vi "dark int time.vi"(8 "error in (no error)":errorcluster, 11 "Settings In":T1) -> (0 "error out":errorcluster, 1 "Stop and Save":bool, 3 "Settings Out":T1)   [LabVIEW 2014, in "AvaSpec.lvlib" / "Dark.lvlib"]
doc: "Determin the integration time to use for the next dark measurement based on how many dark measurements have already been taken and the configuration file."
uses:
  Dark.lvlib
  Settings/Settings.ctl
  Acquisition/Hardware Configuration.ctl
  Libraries/AS-5216-DLL/AVS settings.ctl
  Acquisition/Sphere Indicator.ctl
  Settings/Measurement Type.ctl
  Logging/Logging Configuration.ctl
  Settings/AvaSpec Settings.lvlib
  AvaSpec.lvlib
  Acquisition/AvaSpec Acquisition.lvlib
  Logging/AvaSpec Logging.lvlib
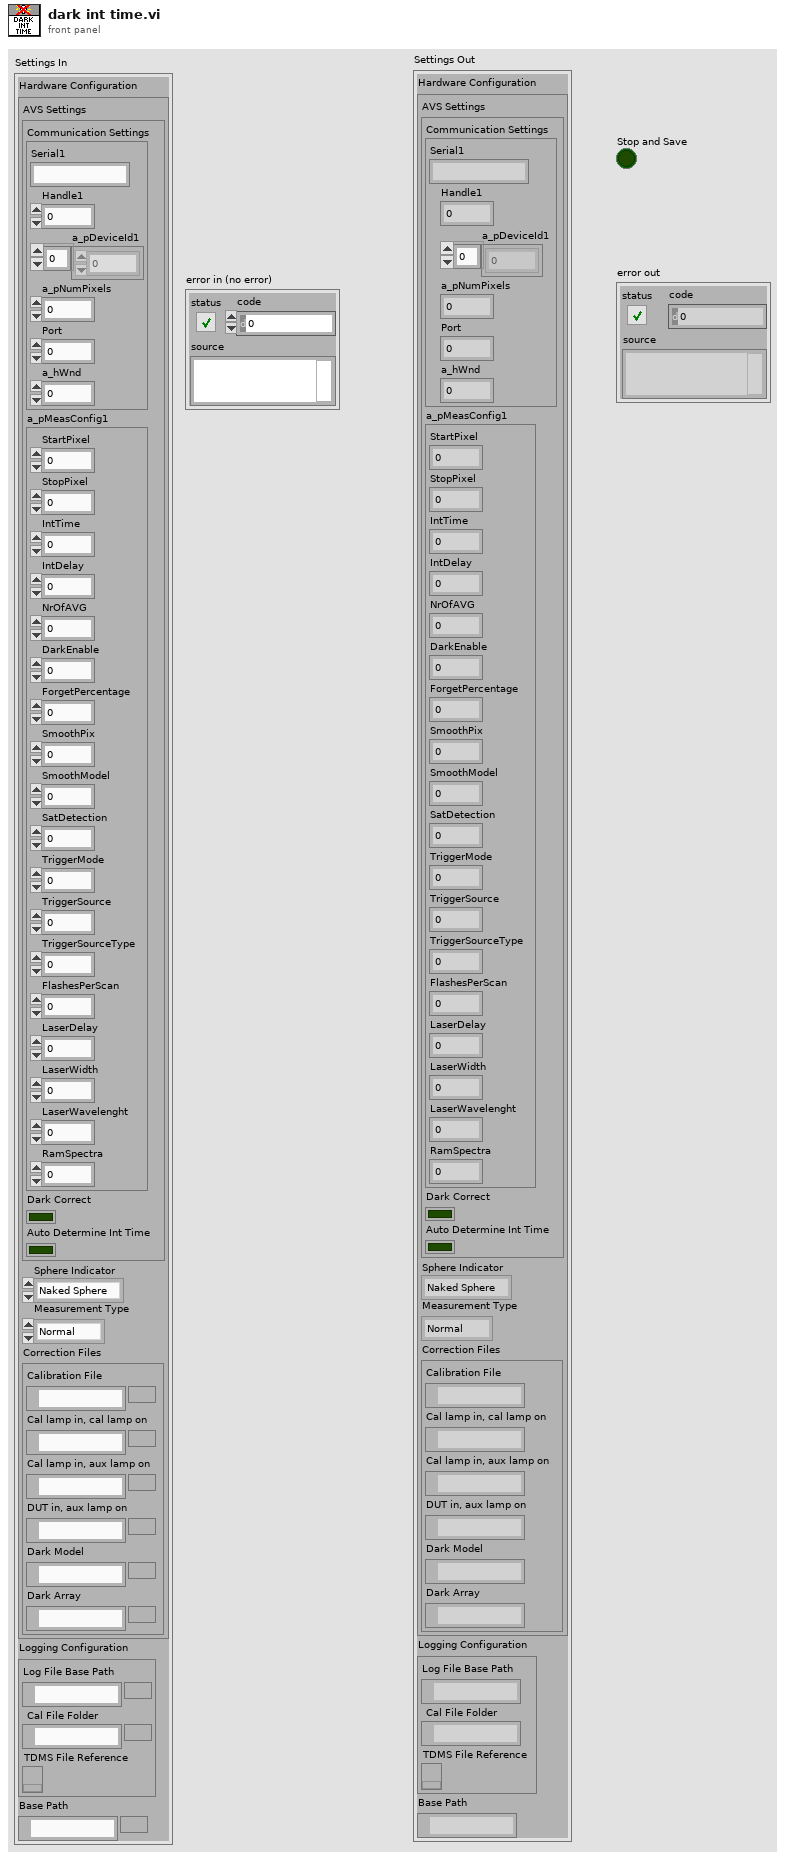
[diagram p1: front panel]
types:
  T1 = typedef "AvaSpec.lvlib/AvaSpec Settings.lvlib/Settings.ctl" = cluster{"Hardware Configuration":T2, "Logging Configuration":T6, "Base Path":path}
  T2 = typedef "AvaSpec.lvlib/AvaSpec Acquisition.lvlib/Hardware Configuration.ctl" = cluster{"AVS Settings":T3, "Sphere Indicator":T4, "Measurement Type":T5, "Correction Files":cluster{"Calibration File":path, "Cal lamp in, cal lamp on":path, "Cal lamp in, aux lamp on":path, "DUT in, aux lamp on":path, "Dark Model":path, "Dark Array":path}}
  T3 = typedef "AvaSpec.lvlib/AVS settings.ctl" = cluster{"Communication Settings":cluster{"Serial1":string, "Handle1":i32, "a_pDeviceId1":u8[], "a_pNumPixels":u16, "Port":i32, "a_hWnd":i32}, "a_pMeasConfig1":cluster{"StartPixel":u16, "StopPixel":u16, "IntTime":sgl, "IntDelay":u32, "NrOfAVG":u32, "DarkEnable":u8, "ForgetPercentage":u8, "SmoothPix":u16, "SmoothModel":u8, "SatDetection":u8, "TriggerMode":u8, "TriggerSource":u8, "TriggerSourceType":u8, "FlashesPerScan":u16, "LaserDelay":u32, "LaserWidth":u32, "LaserWavelenght":sgl, "RamSpectra":u16}, "Dark Correct":bool, "Auto Determine Int Time":bool}
  T4 = typedef "AvaSpec.lvlib/Sphere Indicator.ctl" = enum16{"Naked Sphere", "Insulated Sphere"}
  T5 = typedef "AvaSpec.lvlib/AvaSpec Acquisition.lvlib/Measurement Type.ctl" = enum16{"Normal", "Calibration", "Dark"}
  T6 = typedef "AvaSpec.lvlib/AvaSpec Logging.lvlib/Logging Configuration.ctl" = cluster{"Log File Base Path":path, "Cal File Folder":path, "TDMS File Reference":refnum<k34>}
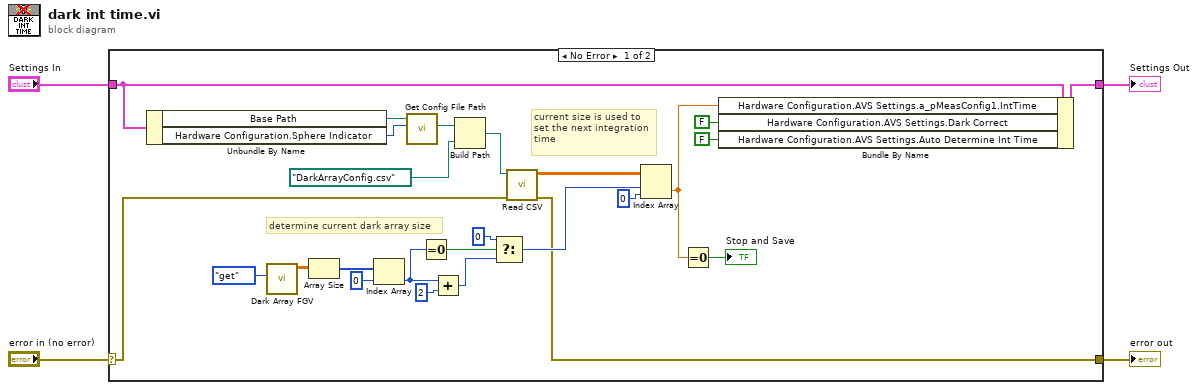
[diagram p0: block diagram]
diagram:
  n1 = case shown="No Error" "error in (no error)" {
    selector: "error in (no error)" -> [w6 w31]
    tunnel: [w5 w31] -> w3
    tunnel: "Settings In" -> [w13 w30]
    tunnel: [w17 w30] -> w1
    frame No Error {
      # "current size is used to\nset the next integration\ntime"
      # "determine current dark array size"
      n2 = Unbundle By Name(w13) -> ("Base Path"=w12:path, "Hardware Configuration.Sphere Indicator"=w9:T4)
      n3 = call "Dark Array FGV.vi"("Control"=enum16{"get", "add", "reset"}."get") -> ("All Dark Measurements Out"=w28:dbl[][])  [unwired: 10 in]
      n4 = Array Size(array=w28) -> (size(s)=w27:i32[])
      n5 = Index Array(array=w27, index=0) -> (element=w22:i32)
      n6 = call "Get Config File Path.vi"("Sphere indicator"=w9, "Base Path"=w12) -> ("Cal File Folder"=w11:path)  [unwired: 7 in, 2 out]
      n7 = Equal To 0?(x=w22) -> (x = 0?=w23:bool)
      n8 = Add(x=w22, y=2) -> (x+y=w21:i32)
      n9 = Build Path(base path=w11, name or relative path=path "DarkArrayConfig.csv" ("file path (dialog if empty)")) -> (appended path=w8:path)
      n10 = Select(t=0, s=w23, f=w21) -> (s? t:f=w19:i32)
      n11 = call "Read CSV.vi"("error in (no error)"=w6, "Path"=w8) -> ("error out"=w5:errorcluster, "all rows"=w7:dbl[][])  [unwired: 7 in, 1 out]
      n12 = Index Array(array=w7, index (row)=w19, index (col)=0 ("disabled index (col)")) -> (element=w16:dbl)
      n13 = Equal To 0?(x=w16) -> (x = 0?=→"Stop and Save":bool)
      n14 = Bundle By Name(cluster=w13, "Hardware Configuration.AVS Settings.a_pMeasConfig1.IntTime"=w16, "Hardware Configuration.AVS Settings.Dark Correct"=FALSE, "Hardware Configuration.AVS Settings.Auto Determine Int Time"=FALSE) -> (w17:T1)
    }
    frame Error {
    }
  }
  "error out" <- w3
  "Settings Out" <- w1
